vi "ULTI_EdgeDetector.vi"(10 "IN (N)":bool, 11 "IN (N+2)":bool) -> (2 "Neg Edge":bool, 3 "Pos Edge":bool)   [LabVIEW 2024]
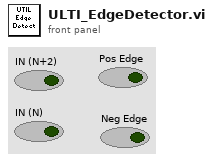
[diagram p1: front panel]
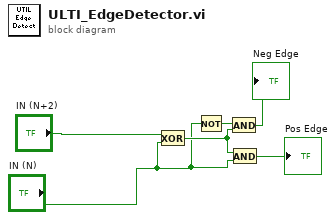
[diagram p0: block diagram]
diagram:
  n1 = Exclusive Or(1:"IN (N)", 2:"IN (N+2)") -> (0:w3:bool)
  n2 = Not(x="IN (N)") -> (.not. x?=w4:bool)
  n3 = And(x=w4, y=w3) -> (x .and. y?=→"Neg Edge":bool)
  n4 = And(x=w3, y="IN (N)") -> (x .and. y?=→"Pos Edge":bool)
